vi "探头面板.vi"() -> ()   [LabVIEW 2017]
uses:
  <vilib>/Platform/TimedLoop/XDataNode/timing_clust.ctl
  <vilib>/Platform/TimedLoop/XDataNode/nitl_modes.ctl
  <vilib>/Platform/TimedLoop/XDataNode/wakeup.ctl
  <vilib>/Platform/TimedLoop/XDataNode/XDataNode.xnode
  <vilib>/Platform/TimedLoop/XDataNode/XDNodeRunTimeDep.lvlib
panel:
  out "报警更新":timestamp format="%<%.3X>T"
  out "测量更新":timestamp format="%<%.3X>T"
  out "remote port":u16 caption="远程端口"
  out "remote address":string caption="远程地址"
  in  "停止按钮":bool
  out "重启":bool
  out "本机IP":string
  out "结构名":string
  in  "端口":u16=60001 min=60000
  in  "报警值":dbl=1.0
  in  "测量值":dbl=0.15
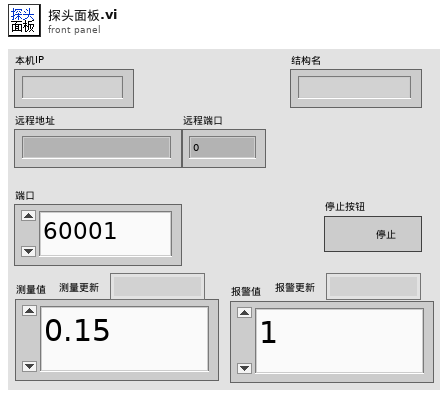
[diagram p1: front panel]
types:
  T1 = typedef "XDNodeRunTimeDep.lvlib/timing_clust.ctl" = cluster{"Expected End [f-1]":u64, "Actual End [f-1]":u64, "Finished Late? [f-1]":bool, "Expected End [i-1]":u64, "Actual End [i-1]":u64, "Finished Late? [i-1]":bool, "Expected Start [i]":u64, "Actual Start [i]":u64, "Expected Start [f]":u64, "Actual Start [f]":u64, "Source Name":string, "Structure Name":string, "Period":i64, "Deadline":i64, "Offset":i64, "Start":i64, "Priority":i32, "Timeout":i32, "Mode":T2, "Wakeup Reason":T3, "Error":errorcluster, "Source Type":string, "Secondary Source Type":string, "Global End Time":u64, "Global Start Time":u64, "Frame Duration":u64, "Iteration Duration":u64, "Assigned CPU":i32, "I/O Scan Engine Mode":u32}
  T2 = typedef "XDNodeRunTimeDep.lvlib/nitl_modes.ctl" = enum32{"No Change", "Process missed periods, maintain original phase", "Discard missed periods, maintain original phase", "Process missed periods, ignore original phase", "Discard missed periods, ignore original phase"}
  T3 = typedef "XDNodeRunTimeDep.lvlib/wakeup.ctl" = enum32{"Normal", "Aborted", "Asynchronous wakeup", "Timing source error", "Timed loop error", "Timeout"}
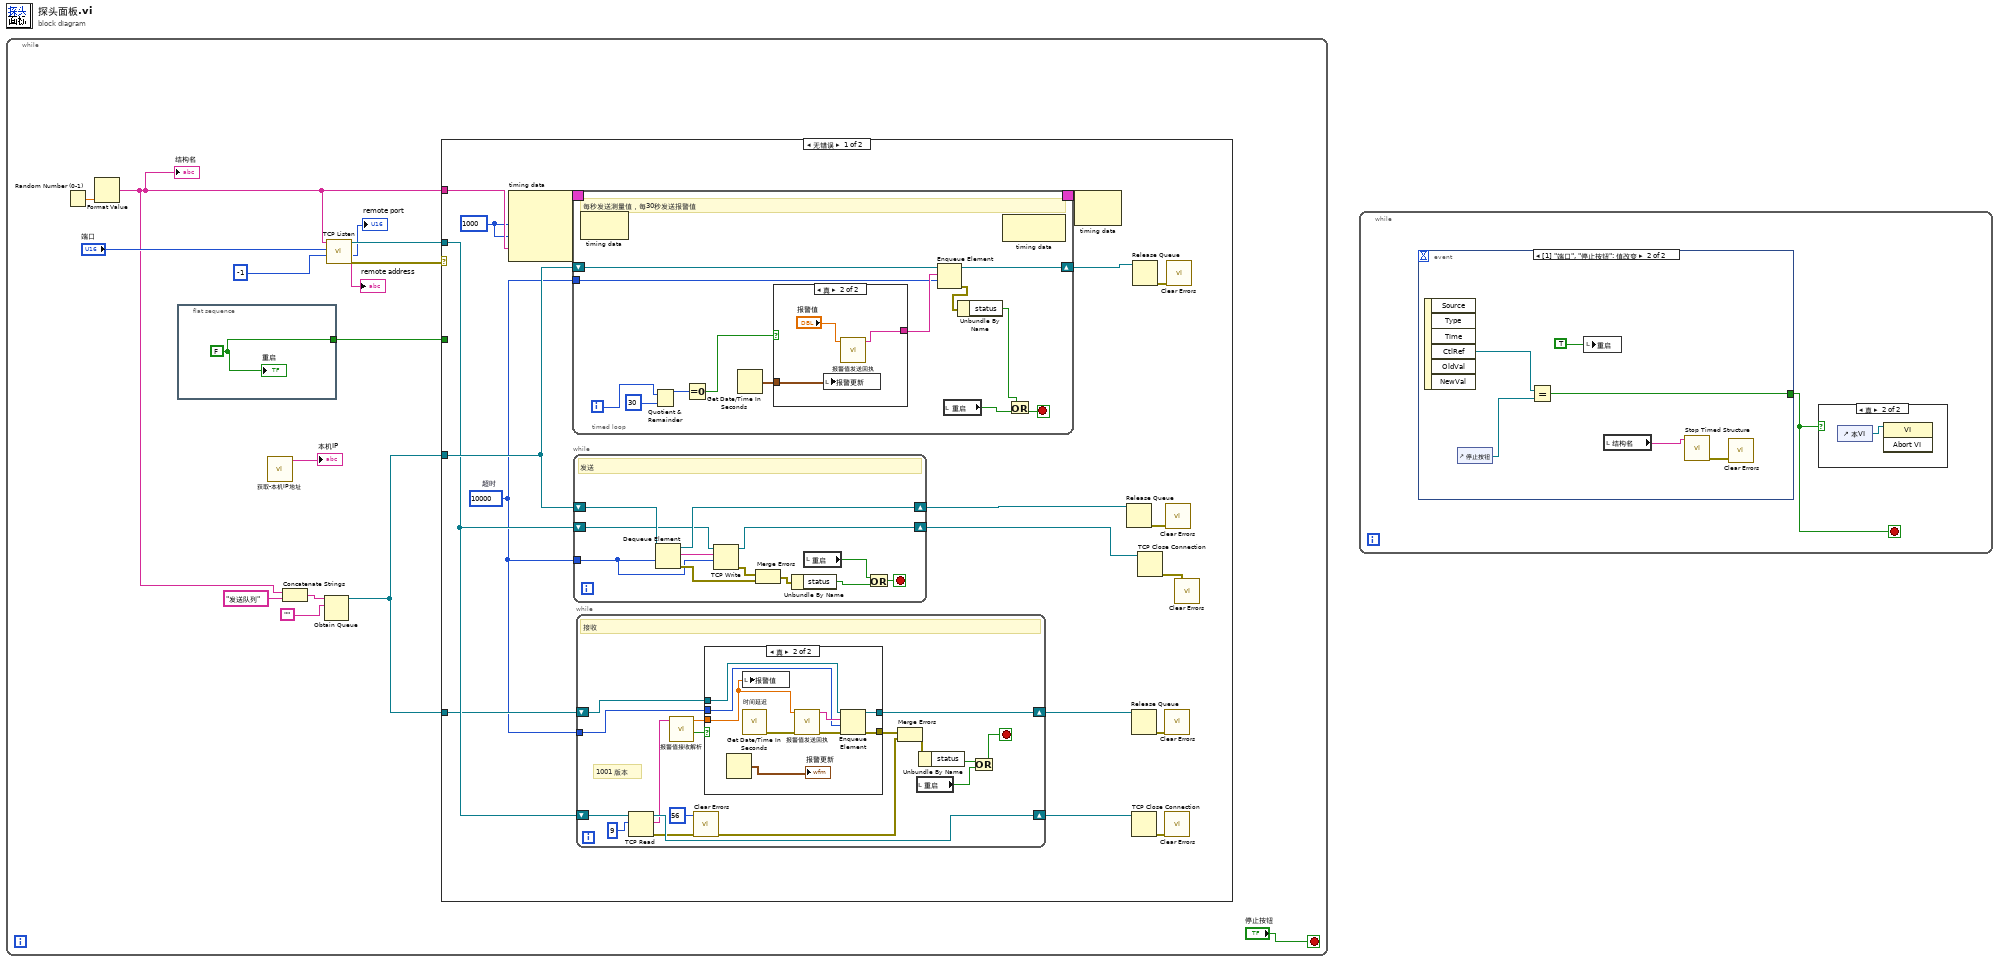
[diagram p0: block diagram]
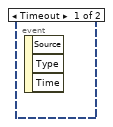
[diagram p3: hidden frame]
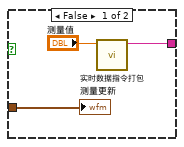
[diagram p5: hidden frame]
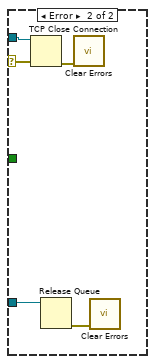
[diagram p6: hidden frame]
diagram:
  n1 = while {
    stop <- "停止按钮" stop-if-true
    n2 = Random Number (0-1)() -> (number: 0 to 1=w6:dbl)
    n3 = Format Value(value (0)=w6) -> (output string=w1:string)  [unwired: 2 in]
    "结构名" <- w1
    n4 = flat-sequence {
      tunnel: [w16] -> w8
      frame #0 {
        w16 = FALSE ("停止按钮")
        "重启" <- w16
      }
    }
    n5 = call "获取-本机IP地址.vi"() -> ("本机IP"=→"本机IP":string)  [unwired: 11 in]
    n6 = Concatenate Strings(w1, "发送队列" ("名称（未命名）")) -> (w2:string)
    n7 = Obtain Queue(name (unnamed)=w2, element data type="") -> (queue out=w13:refnum<queue>)  [unwired: 3 in, 2 out]
    n8 = call <vilib>:"TCP Listen.vi"("timeout ms (wait forever: -1)"=-1 ("超时毫秒(25000)"), "port"="端口", "service name"=w1) -> ("error out"=w10:errorcluster, "remote port"=→"remote port":u16, "remote address"=→"remote address":string, "connection ID"=w11:refnum<k5>)  [unwired: 4 in, 1 out]
    n9 = case shown="无错误" w10 {
      selector: w10 -> [_ w105]
      tunnel: w1 -> [w32 _]
      tunnel: w13 -> [w31 w102]
      tunnel: w11 -> [w26 w104]
      tunnel: w13 -> [w25 _]
      tunnel: w8 -> [_ _]
      frame No Error {
        w17 = i64 1000 ("周期")
        w24 = 10000  # 超时
        n10 = node-c288(w17, w17, w32) -> (w34:T1)  [unwired: 1 in]
        n11 = timed-loop {
          timing: w34 -> [_]
          timing-out: [_] -> w33
          shift-right: [w84] -> w30
          shift-left: w31 -> [w86]
          tunnel: w24 -> [w83]
          i -> [w82]
          stop <- w76 stop-if-true
          # "每秒发送测量值，每30秒发送报警值"
          n12 = node-c288() -> ()  [unwired: 1 in, 1 out]
          n13 = Quotient & Remainder(x=w82, y=30) -> (x-y*floor(x/y)=w80:i32)  [unwired: 1 out]
          n14 = Equal To 0?(x=w80) -> (x = 0?=w79:bool)
          n15 = Get Date/Time In Seconds() -> (seconds since 1Jan1904=w74:timestamp)
          n16 = case shown="真" w79 {
            tunnel: [w88 w91] -> w85
            tunnel: w74 -> [w87 w90]
            frame False {
              n17 = call "实时数据指令打包.vi"("测量值"="测量值") -> ("完整输出"=w88:string)  [unwired: 9 in, 1 out]
              "测量更新" <- w87
            }
            frame True {
              n18 = local write "报警更新"(w90) -> ()
              n19 = call "报警值发送回执.vi"("限值"="报警值") -> ("指令输出"=w91:string)  [unwired: 9 in, 1 out]
            }
          }
          n20 = Enqueue Element(queue=w86, element=w85, timeout in ms (-1)=w83) -> (queue out=w84:refnum<queue>, error out=w78:errorcluster)  [unwired: 1 in, 1 out]
          n21 = local read "重启"() -> (w77:bool)
          n22 = Unbundle By Name(w78) -> ("status"=w75:bool)
          n23 = node-c288() -> ()  [unwired: 1 in, 1 out]
          n24 = Or(x=w75, y=w77) -> (x .or. y?=w76:bool)
        }
        n25 = while {
          shift-right: [w72] -> w28
          shift-left: w31 -> [w73]
          tunnel: w24 -> [w68]
          shift-right: [w65] -> w23
          shift-left: w26 -> [w70]
          stop <- w63 stop-if-true
          # "发送"
          n26 = Dequeue Element(queue=w73, timeout in ms (-1)=w68) -> (queue out=w72:refnum<queue>, element=w69:string, error out=w71:errorcluster)  [unwired: 1 in, 1 out]
          n27 = TCP Write(connection ID=w70, data in=w69, 9:w68) -> (connection ID out=w65:refnum<k5>, error out=w66:errorcluster)  [unwired: 1 in, 1 out]
          n28 = Merge Errors(w66, w71) -> (w67:errorcluster)
          n29 = Unbundle By Name(w67) -> ("status"=w64:bool)
          n30 = local read "重启"() -> (w62:bool)
          n31 = Or(x=w62, y=w64) -> (x .or. y?=w63:bool)
        }
        n32 = while {
          shift-right: [w46] -> w22
          shift-left: w26 -> [w47]
          shift-right: [w48] -> w18
          shift-left: w25 -> [w49]
          tunnel: w24 -> [w35]
          stop <- w37 stop-if-true
          # "1001 版本"
          # "接收"
          n33 = TCP Read(connection ID=w47, bytes to read=9 ("读取的字节")) -> (connection ID out=w46:refnum<k5>, data out=w41:string, error out=w44:errorcluster)  [unwired: 3 in]
          n34 = call "报警值接收解析.vi"("完整输入"=w41) -> ("有效数据？"=w40:bool, "限值"=w39:dbl)  [unwired: 9 in]
          n35 = call <vilib>:"Clear Errors.vi"("error in (no error)"=w44, "specific error code to clear (0: all)"=56) -> ("error out"=w42:errorcluster)  [unwired: 4 in, 1 out]
          n36 = case shown="真" w40 {
            tunnel: [_ w61] -> w51
            tunnel: w49 -> [w52 w60]
            tunnel: [w52 w59] -> w48
            tunnel: w39 -> [_ w57]
            tunnel: w35 -> [_ w55]
            frame False {
            }
            frame True {
              n37 = Get Date/Time In Seconds() -> (seconds since 1Jan1904=→"报警更新":timestamp)
              n38 = local write "报警值"(w57) -> ()
              n39 = call "时间延迟"() -> ("error out"=w58:errorcluster)  [unwired: 11 in]
              n40 = call "报警值发送回执.vi"("错误 i"=w58, "限值"=w57) -> ("错误 o"=w54:errorcluster, "指令输出"=w56:string)  [unwired: 8 in]
              n41 = Enqueue Element(queue=w60, element=w56, timeout in ms (-1)=w55, error in (no error)=w54) -> (queue out=w59:refnum<queue>, error out=w61:errorcluster)  [unwired: 1 out]
            }
          }
          n42 = Merge Errors(w51, w42) -> (w50:errorcluster)
          n43 = local read "重启"() -> (w36:bool)
          n44 = Unbundle By Name(w50) -> ("status"=w38:bool)
          n45 = Or(x=w38, y=w36) -> (x .or. y?=w37:bool)
        }
        n46 = node-c288(w33) -> ()  [unwired: 1 out]
        n47 = Release Queue(queue=w28) -> (error out=w27:errorcluster)  [unwired: 2 in, 2 out]
        n48 = Release Queue(queue=w18) -> (error out=w19:errorcluster)  [unwired: 2 in, 2 out]
        n49 = TCP Close Connection(connection ID=w22) -> (error out=w20:errorcluster)  [unwired: 2 in, 1 out]
        n50 = Release Queue(queue=w30) -> (error out=w29:errorcluster)  [unwired: 2 in, 2 out]
        n51 = TCP Close Connection(connection ID=w23) -> (error out=w21:errorcluster)  [unwired: 2 in, 1 out]
        n52 = call <vilib>:"Clear Errors.vi"("error in (no error)"=w19) -> ()  [unwired: 5 in, 2 out]
        n53 = call <vilib>:"Clear Errors.vi"("error in (no error)"=w20) -> ()  [unwired: 5 in, 2 out]
        n54 = call <vilib>:"Clear Errors.vi"("error in (no error)"=w27) -> ()  [unwired: 5 in, 2 out]
        n55 = call <vilib>:"Clear Errors.vi"("error in (no error)"=w29) -> ()  [unwired: 5 in, 2 out]
        n56 = call <vilib>:"Clear Errors.vi"("error in (no error)"=w21) -> ()  [unwired: 5 in, 2 out]
      }
      frame Error {
        n57 = TCP Close Connection(connection ID=w104, error in (no error)=w105) -> (error out=w103:errorcluster)  [unwired: 1 in, 1 out]
        n58 = Release Queue(queue=w102) -> (error out=w101:errorcluster)  [unwired: 2 in, 2 out]
        n59 = call <vilib>:"Clear Errors.vi"("error in (no error)"=w103) -> ()  [unwired: 5 in, 2 out]
        n60 = call <vilib>:"Clear Errors.vi"("error in (no error)"=w101) -> ()  [unwired: 5 in, 2 out]
      }
    }
  }
  n61 = while {
    stop <- w106 stop-if-true
    n62 = event shown="[1] \"端口\", \"停止按钮\": 值改变" {
      selector: _ -> [_ _]
      dyn-events: _ -> [_ _]
      timeout: _ -> [_ _]
      tunnel: [_ w110] -> w106
      event Timeout {
        n63 = event-data() -> ()  [unwired: 1 in, 3 out]
      }
      event "端口", "停止按钮": Value Change {
        n64 = event-data() -> ("CtlRef"=w111:refnum<vi>)  [unwired: 1 in, 5 out]
        n65 = control-ref of="停止按钮"() -> (w112:refnum<vi>)
        n66 = Equal?(x=w111, y=w112) -> (x = y?=w110:bool)
        n67 = local write "重启"(TRUE ("停止按钮")) -> ()
        n68 = local read "结构名"() -> (w109:string)
        n69 = call <vilib>:"Stop Timed Structure.vi"("name"=w109) -> ("error out"=w108:errorcluster)  [unwired: 10 in]
        n70 = call <vilib>:"Clear Errors.vi"("error in (no error)"=w108) -> ()  [unwired: 5 in, 2 out]
      }
    }
    n71 = case shown="真" w106 {
      frame False {
      }
      frame True {
        n72 = control-ref of="本VI"() -> (w107:refnum<vi>)
        n73 = invoke class="VI" method="Abort VI"(reference=w107) -> ()  [unwired: 2 in, 3 out]
      }
    }
  }
